vi "Scroll Text.vi"(8 "error in (no error)":errorcluster, 11 "String":string) -> (0 "error out":errorcluster, 3 "At End":bool)   [LabVIEW 2015]
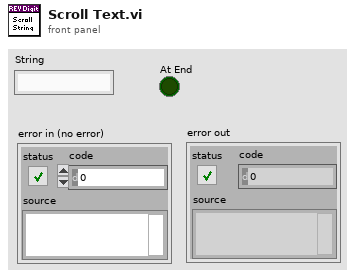
[diagram p1: front panel]
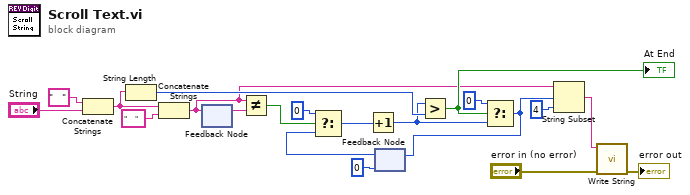
[diagram p0: block diagram]
diagram:
  n1 = Concatenate Strings("   " ("string"), "String") -> (w2:string)
  n2 = String Length(string=w2) -> (length=w15:i32)
  n3 = Concatenate Strings(w2, "    " ("string")) -> (w9:string)
  n4 = feedback-in #1(w9) -> ()
  n5 = feedback #1() -> (w20:string)  [unwired: 1 in]
  n6 = Not Equal?(x=w9, y=w20) -> (x != y?=w19:bool)
  n7 = feedback #2(0) -> (w17:i32)
  n8 = Select(t=0, s=w19, f=w17) -> (s? t:f=w16:i32)
  n9 = Increment(x=w16) -> (x+1=w12:i32)
  n10 = Greater?(x=w12, y=w15) -> (0:w14:bool)
  "At End" <- w14
  n11 = Select(t=0, s=w14, f=w12) -> (s? t:f=w8:i32)
  n12 = feedback-in #2(w8) -> ()
  n13 = String Subset(string=w9, offset (0)=w8, length (rest)=4 ("length (rest)")) -> (substring=w5:string)
  n14 = call "Write String.vi"("error in (no error)"="error in (no error)", "String"=w5) -> ("error out"=→"error out":errorcluster)  [unwired: 9 in]
